vi "Populate Bookmarks View.vi"(8 "Error In":errorcluster, 11 "State In":T1) -> (0 "Error Out":errorcluster, 3 "State Out":T1)   [LabVIEW 2017, in "Graveyard.lvlib"]
uses:
  Graveyard.lvlib
  State.ctl
  VI Bookmark.ctl
  VI Information.ctl
  Application Information.ctl
  Bookmarks Views.ctl
  Eulogy/Public/Bookmarks.ctl
  Eulogy/Eulogy.lvlib
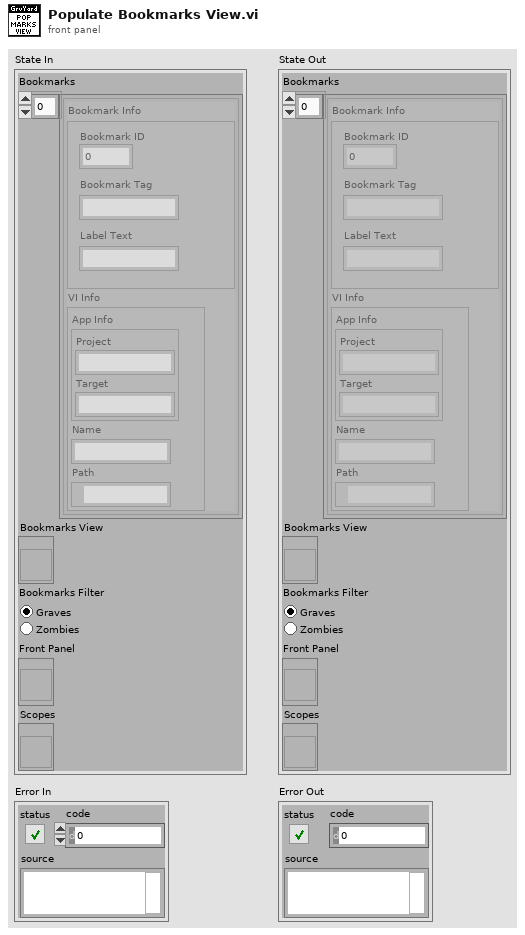
[diagram p1: front panel]
types:
  T1 = typedef "Graveyard.lvlib/State.ctl" = cluster{"Bookmarks":T2[], "Bookmarks View":refnum<vi>, "Bookmarks Filter":T5, "Front Panel":refnum<vi>, "Scopes":refnum<vi>}
  T2 = typedef "Graveyard.lvlib/VI Bookmark.ctl" = cluster{"Bookmark Info":cluster{"Bookmark ID":u32, "Bookmark Tag":string, "Label Text":string}, "VI Info":T3}
  T3 = typedef "Graveyard.lvlib/VI Information.ctl" = cluster{"App Info":T4, "Name":string, "Path":path}
  T4 = typedef "Graveyard.lvlib/Application Information.ctl" = cluster{"Project":string, "Target":string}
  T5 = typedef "Graveyard.lvlib/Bookmarks Views.ctl" = enum32{"Graves", "Zombies"}
  T6 = enum8{"Enabled", "Disabled", "Disabled and Grayed Out"}
  T7 = typedef "Eulogy.lvlib/Bookmarks.ctl" = enum16{"RIP", "Zombie"}
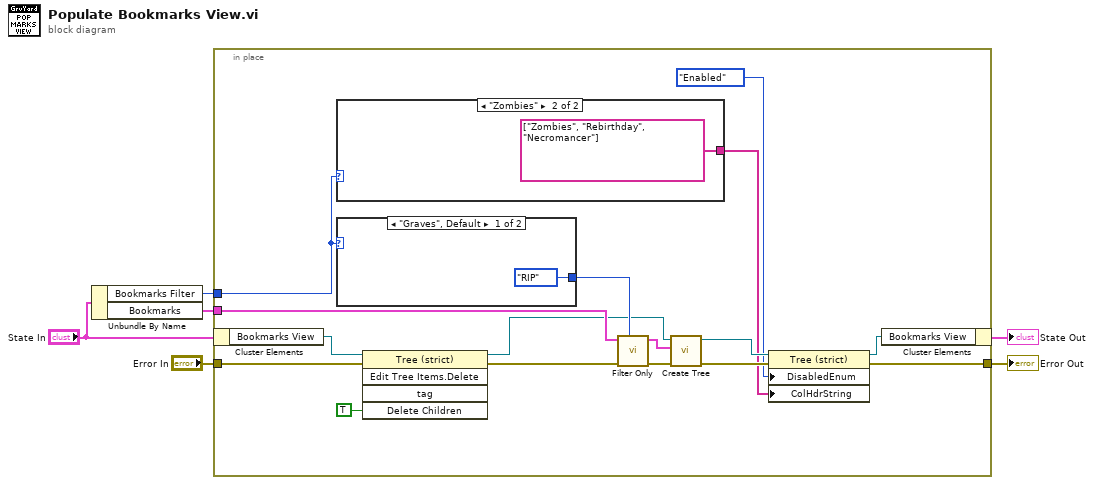
[diagram p0: block diagram]
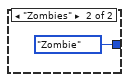
[diagram p2: hidden frame]
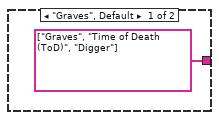
[diagram p3: hidden frame]
diagram:
  n1 = Unbundle By Name("State In") -> ("Bookmarks Filter"=w2:T5, "Bookmarks"=w1:T2[])
  n2 = in-place {
    in-place-border: "Error In" -> [w22]
    in-place-border: [w20] -> w4
    in-place-border: w2 -> [w17]
    in-place-border: w1 -> [w14]
    n3 = in-place-cluster #1("State In") -> ("Bookmarks View"=w9:refnum<vi>)
    n4 = case shown="\"Zombies\"" w17 {
      tunnel: [string[] ["Graves", "Time of Death (ToD)", "Digger"] string[] ["Zombies", "Rebirthday", "Necromancer"]] -> w16
      frame "Graves", Default {
      }
      frame "Zombies" {
      }
    }
    n5 = case shown="\"Graves\", Default" w17 {
      tunnel: [Bookmarks."RIP" ("Bookmark") Bookmarks."Zombie" ("Bookmark")] -> w12
      frame "Graves", Default {
      }
      frame "Zombies" {
      }
    }
    n6 = invoke class="Tree (strict)" method="Edit Tree Items.Delete"(reference=w9, error in=w22, "Delete Children"=TRUE ("Delete Children?")) -> (reference out=w7:refnum<vi>, error out=w10:errorcluster)  [unwired: 2 in, 3 out]
    n7 = call "Filter Only.vi"("Bookmark"=w12, "Error In"=w10, "VI Bookmarks"=w14) -> ("Error Out"=w13:errorcluster, "Graves"=w11:T2[])  [unwired: 7 in]
    n8 = call "Create Tree.vi"("Error In"=w13, "Eulogy Bookmarks"=w11, "TreeControl In"=w7) -> ("Error Out"=w21:errorcluster, "TreeControl Out"=w19:refnum<vi>)  [unwired: 7 in]
    n9 = property class="Tree (strict)"(reference=w19, error in=w21, "DisabledEnum"=T6."Enabled" ("Disabled"), "ColHdrString"=w16) -> (reference out=w18:refnum<vi>, error out=w20:errorcluster)
    n10 = in-place-cluster #1("Bookmarks View"=w18) -> (→"State Out":T1)
  }
  "Error Out" <- w4
